vi "create_standards.vi"   [LabVIEW 2017]
doc: "reads the Standards.ini and creates the standards objects"
uses:
  Classes/Standard/Standard.lvclass
  <vilib>/Utility/config.llb/Read Key (String).vi
  <vilib>/Utility/config.llb/Read Key (Double).vi
  <vilib>/Utility/config.llb/NI_LVConfig.lvlib
types:
  T1 = typedef "NI_LVConfig.lvlib/Config Data RefNum.ctl" = refnum<k1>
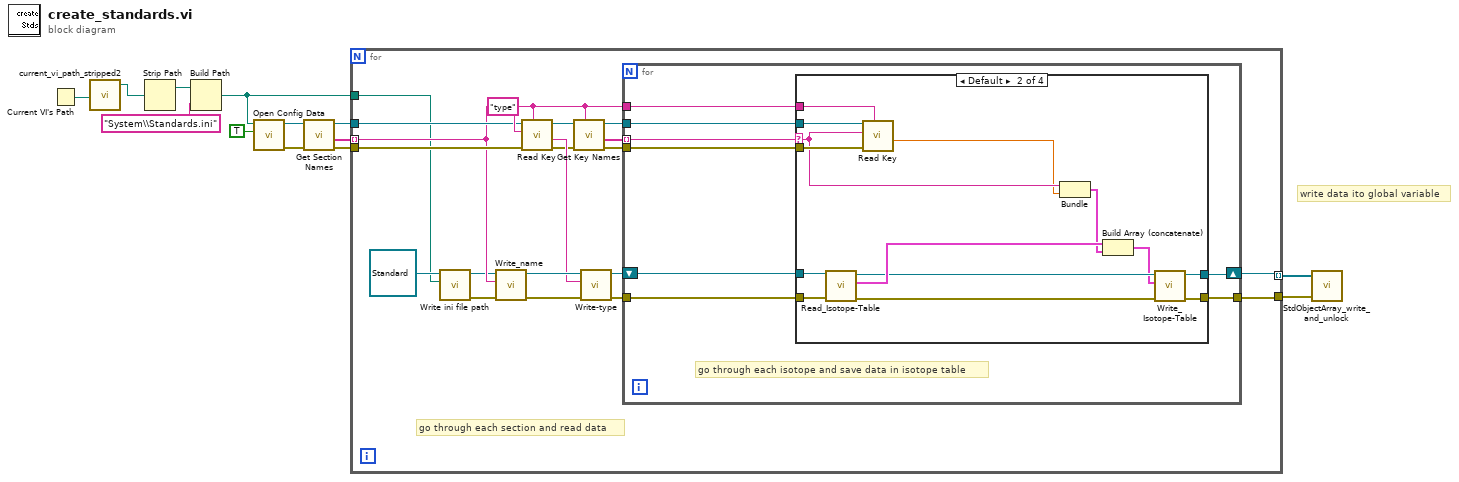
[diagram p0: block diagram]
diagram:
  # "write data ito global variable"
  n1 = Current VI's Path() -> (path=w8:path)
  n2 = call "current_vi_path_stripped2.vi"("current VI Path"=w8) -> ("current VI Path stripped out"=w3:path)  [unwired: 3 in, 1 out]
  n3 = Strip Path(path=w3) -> (stripped path=w4:path)  [unwired: 1 out]
  n4 = Build Path(base path=w4, name or relative path="System\\Standards.ini") -> (appended path=w1:path)
  n5 = call <vilib>:"Open Config Data.vi"("create file if necessary (T)"=TRUE, "configuration file path"=w1) -> ("error out"=w9:errorcluster, "refnum"=w10:T1)  [unwired: 7 in, 1 out]
  n6 = call <vilib>:"Get Section Names.vi"("error in (no error)"=w9, "refnum"=w10) -> ("error out"=w13:errorcluster, "section names"=w11:string[], "refnum out"=w12:T1)  [unwired: 7 in]
  n7 = for {
    tunnel: w11 -> [w18] mode=indexing
    tunnel: w12 -> [w20]
    tunnel: w13 -> [w19]
    tunnel: [w22] -> w5 mode=indexing
    tunnel: [w21] -> w2
    tunnel: w1 -> [w14]
    # "go through each section and read data"
    n8 = call-dynamic "Write ini file path.vi"("ini file path"=w14, "Standard in"=refnum<class "Standard.lvclass"> refnum ("Standard.lvclass")) -> ("error out"=w15:errorcluster, "Standard out"=w16:refnum<class "Standard.lvclass">)  [unwired: 8 in]
    n9 = call-dynamic "Write_name.vi"("error in (no error)"=w15, "standard name"=w18, "Standard in"=w16) -> ("error out"=w32:errorcluster, "Standard out"=w33:refnum<class "Standard.lvclass">)  [unwired: 7 in]
    n10 = call-poly <vilib>:"Read Key.vi"("section"=w18, "error in (no error)"=w19, "key"="type", "refnum"=w20) -> ("error out"=w28:errorcluster, "value"=w30:string, "refnum out"=w29:T1)  [unwired: 4 in, 1 out]
    n11 = call <vilib>:"Get Key Names.vi"("section"=w18, "error in (no error)"=w28, "refnum"=w29) -> ("error out"=w26:errorcluster, "key names"=w25:string[], "refnum out"=w27:T1)  [unwired: 5 in, 1 out]
    n12 = call-dynamic "Write-type.vi"("error in (no error)"=w32, "type"=w30, "Standard in"=w33) -> ("error out"=w23:errorcluster, "Standard out"=w24:refnum<class "Standard.lvclass">)  [unwired: 7 in]
    n13 = for {
      tunnel: w27 -> [w41]
      tunnel: w26 -> [w40]
      tunnel: w25 -> [w34] mode=indexing
      tunnel: w23 -> [w38]
      shift-right: [w36] -> w22
      shift-left: w24 -> [w39]
      tunnel: w18 -> [w37]
      tunnel: [w35] -> w21
      # "go through each isotope and save data in isotope table"
      n14 = case shown="Default" w34 {
        selector: w34 -> [_ w45 _ _]
        tunnel: w41 -> [_ w55 _ _]
        tunnel: w40 -> [_ w53 _ _]
        tunnel: w39 -> [w43 w57 w59 w61]
        tunnel: w38 -> [w42 w56 w58 w60]
        tunnel: w37 -> [_ w54 _ _]
        tunnel: [w43 w47 w59 w61] -> w36
        tunnel: [w42 w46 w58 w60] -> w35
        frame "pipettes" {
          # "do not process that key"
        }
        frame Default {
          n15 = call-dynamic "Read_Isotope-Table.vi"("error in (no error)"=w56, "Standard in"=w57) -> ("error out"=w49:errorcluster, "Isotope Table"=w52:cluster{"isotope":string, "amount cc":dbl}[], "Standard out"=w50:refnum<class "Standard.lvclass">)  [unwired: 7 in]
          n16 = call-poly <vilib>:"Read Key.vi"("section"=w54, "error in (no error)"=w53, "key"=w45, "refnum"=w55) -> ("value"=w44:dbl)  [unwired: 4 in, 3 out]
          n17 = Bundle(w45, "value"=w44) -> (w51:cluster{string, "value":dbl})  [unwired: 1 in]
          n18 = Build Array (concatenate)(w52, w51) -> (w48:cluster{"isotope":string, "value":dbl}[])
          n19 = call-dynamic "Write_Isotope-Table.vi"("error in (no error)"=w49, "Isotope Table"=w48, "Standard in"=w50) -> ("error out"=w46:errorcluster, "Standard out"=w47:refnum<class "Standard.lvclass">)  [unwired: 7 in]
        }
        frame "name" {
          # "do not process that key"
        }
        frame "type" {
          # "do not process that key"
        }
      }
    }
  }
  n20 = call "StdObjectArray_write_and_unlock.vi"("error in (no error)"=w2, "StandardObjects"=w5) -> ()  [unwired: 9 in, 1 out]
